vi "Untitled 1.vi"() -> ()   [LabVIEW 2025]
panel:
  out "Array":dbl[](array[numeric])
  out "Waveform Graph":dbl[](graph)
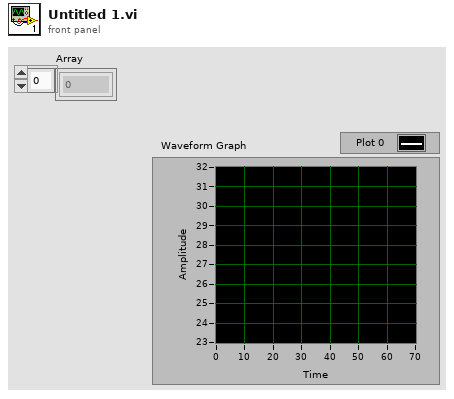
[diagram p1: front panel]
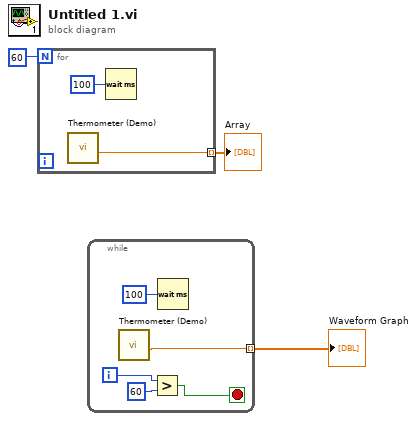
[diagram p0: block diagram]
diagram:
  n1 = for {
    N: 60 -> [_]
    tunnel: [w4] -> w1 mode=indexing
    n2 = call "Thermometer (Demo).vi"() -> ("Temperature Value"=w4:dbl)  [unwired: 11 in]
    n3 = Wait (ms)(milliseconds to wait=u32 100) -> ()  [unwired: 1 out]
  }
  "Array" <- w1
  n4 = while {
    tunnel: [w9] -> w2 mode=indexing
    i -> [w8]
    stop <- w6 stop-if-true
    n5 = call "Thermometer (Demo).vi"() -> ("Temperature Value"=w9:dbl)  [unwired: 11 in]
    n6 = Greater?(x=w8, y=60) -> (0:w6:bool)
    n7 = Wait (ms)(milliseconds to wait=u32 100) -> ()  [unwired: 1 out]
  }
  "Waveform Graph" <- w2
